vi "柱塞泵调试界面.vi"() -> ()   [LabVIEW 2016, in "质控单元.lvlib"]
uses:
  <vilib>/Utility/miscctls.llb/LVPointTypeDef.ctl
  <vilib>/Analysis/6fits.llb/Curve Fitting Criteria.ctl
  <vilib>/Utility/config.llb/Write Key (U32).vi
  <vilib>/Analysis/NI_AALPro.lvlib
  <vilib>/Utility/config.llb/NI_LVConfig.lvlib
panel:
  in  "B 5":dbl caption="B5"
  in  "K 5":dbl caption="K5"
  in  "柱塞泵5":bool
  out "关闭 2":bool=TRUE
  in  "柱塞泵4":bool
  in  "柱塞泵3":bool
  in  "柱塞泵2":bool
  in  "柱塞泵1":bool
  in  "注出体积选择":u16(ring) items=["0.1mL", "0.3mL", "0.5mL", "0.8mL", "1.0mL"]
  out "线性值":T1
  in  "读取":bool
  in  "写入":bool
  in  "柱塞泵枚举":enum16{"氨氮", "总磷", "总氮", "CODMn", "CODCr"}(ring)
  in  "启用计算":bool
  in  "标准体积 2":dbl
  in  "标准体积 3":dbl
  in  "实际体积 1":dbl
  in  "实际体积 2":dbl
  in  "实际体积 3":dbl
  in  "标准体积 4":dbl
  in  "实际体积 4":dbl
  in  "标准体积 5":dbl
  in  "实际体积 5":dbl
  in  "标准体积 1":dbl
  out "拟合方程":string
  out "r^2":dbl format="%_6g"
  in  "B 4":dbl caption="B4"
  in  "K 4":dbl caption="K4"
  in  "B 3":dbl caption="B3"
  in  "K 3":dbl caption="K3"
  in  "B 2":dbl caption="B2"
  in  "K 2":dbl caption="K2"
  in  "B":dbl caption="B1"
  in  "K":dbl caption="K1"
  in  "关闭":bool
  # "柱塞泵手动调试计算界面"
  # "柱塞泵启动控制"
  # "柱塞泵5点线性计算"
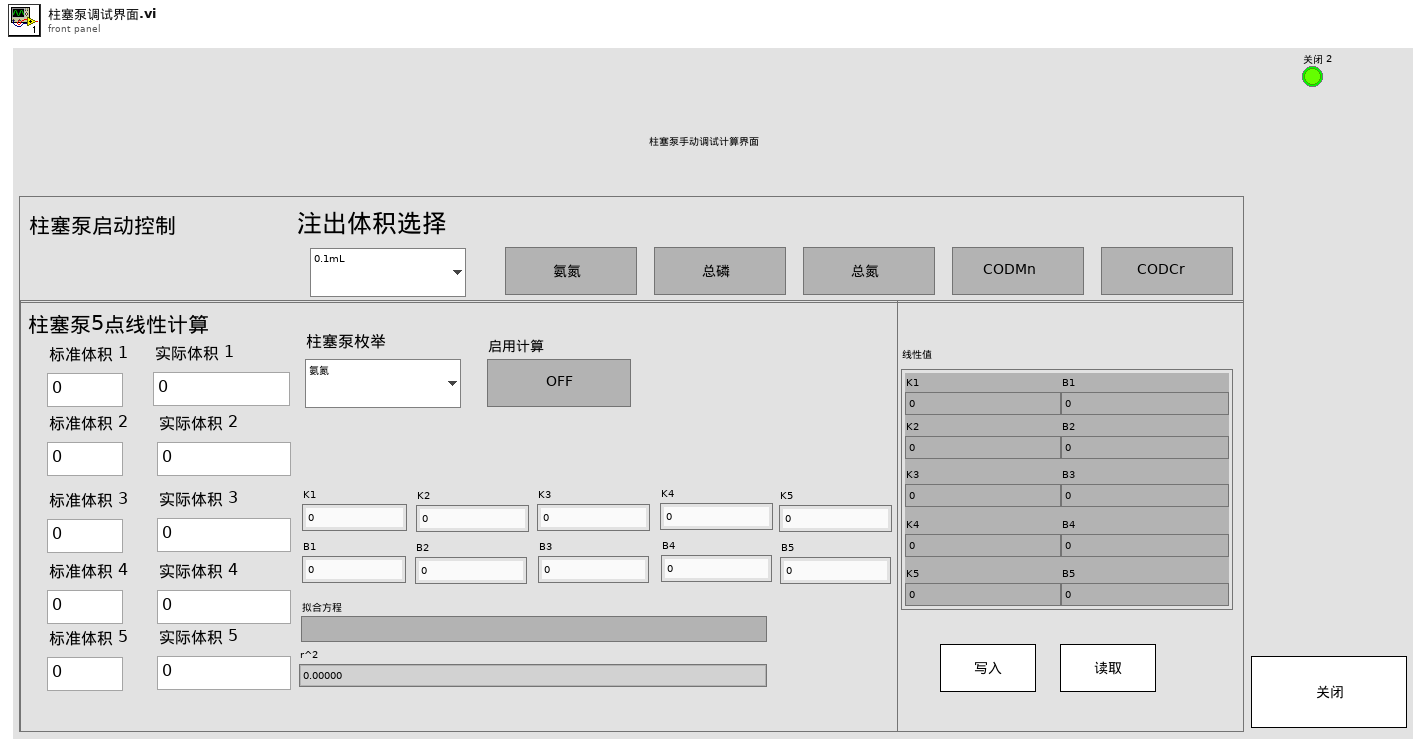
[diagram p1: front panel]
types:
  T1 = cluster{"K1":sgl, "B1":sgl, "K2":sgl, "B2":sgl, "K3":sgl, "B3":sgl, "K4":sgl, "B4":sgl, "K5":sgl, "B5":sgl}
  T2 = typedef "LVPointTypeDef.ctl" = cluster{"Horizontal":i16, "Vertical":i16}
  T3 = cluster{"氨氮":u8, "总磷":u8, "总氮":u8, "CODMn":u8, "CODCr":u8}
  T4 = typedef "NI_LVConfig.lvlib/Config Data RefNum.ctl" = refnum<k1>
  T5 = cluster{"数值":sgl, "数值":sgl, "数值":sgl, "数值":sgl, "数值":sgl, "数值":sgl, "数值":sgl, "数值":sgl, "数值":sgl, "数值":sgl}
  T6 = typedef "NI_AALPro.lvlib/Curve Fitting Criteria.ctl" = u16
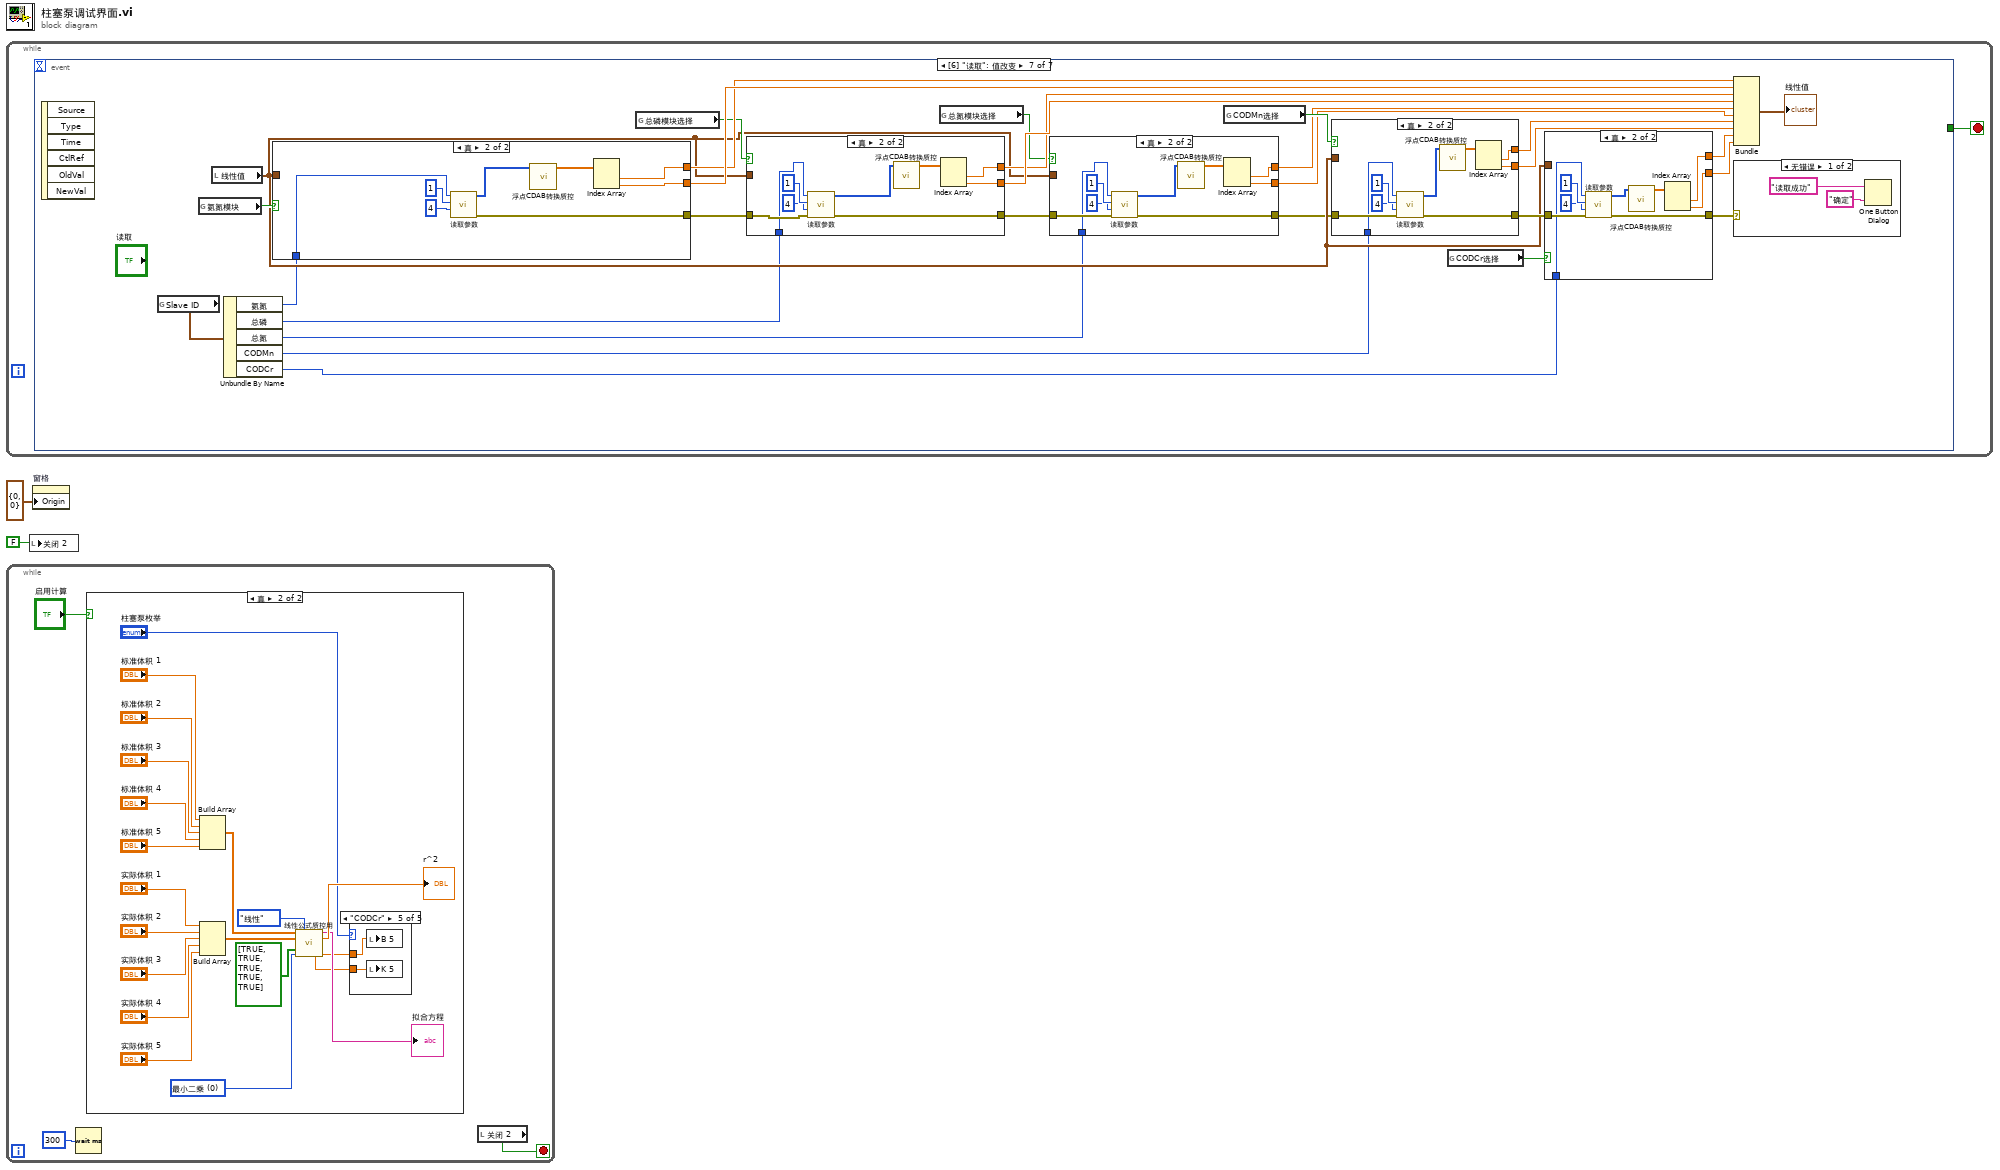
[diagram p0: block diagram]
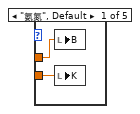
[diagram p3: hidden frame]
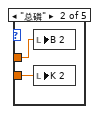
[diagram p4: hidden frame]
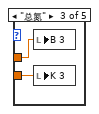
[diagram p5: hidden frame]
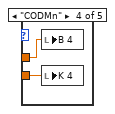
[diagram p6: hidden frame]
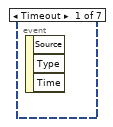
[diagram p7: hidden frame]
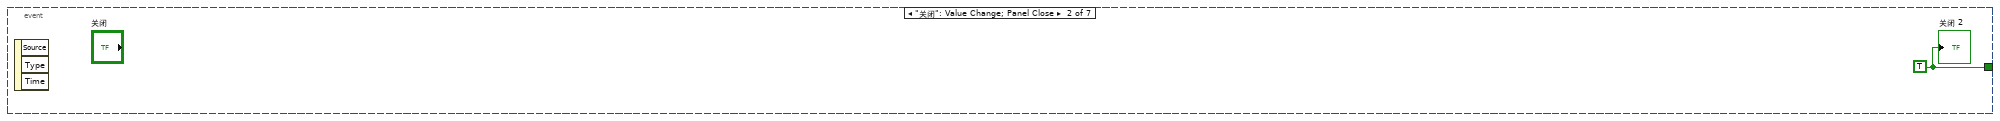
[diagram p8: hidden frame]
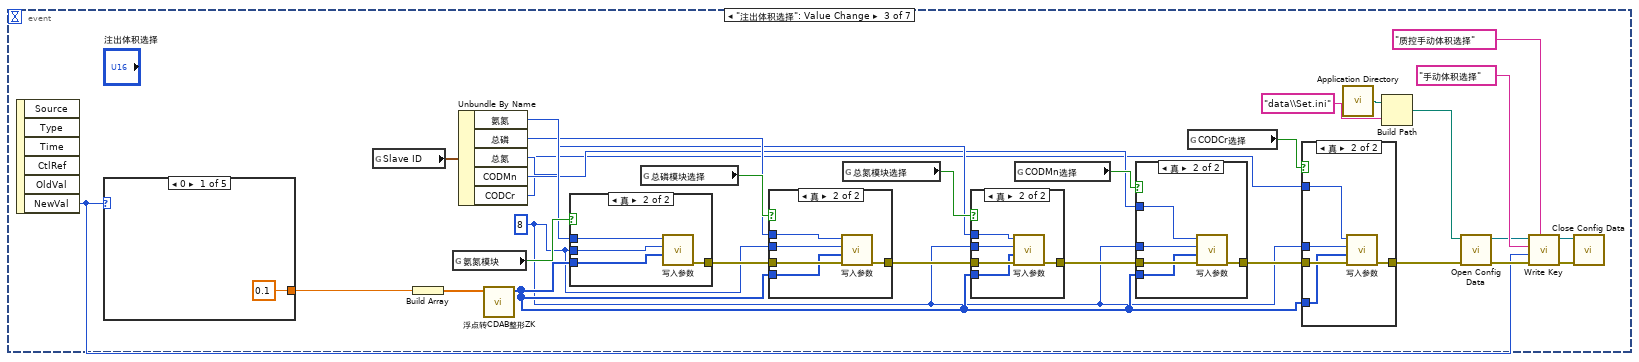
[diagram p9: hidden frame]
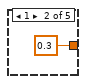
[diagram p15: hidden frame]
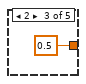
[diagram p16: hidden frame]
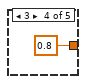
[diagram p17: hidden frame]
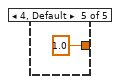
[diagram p18: hidden frame]
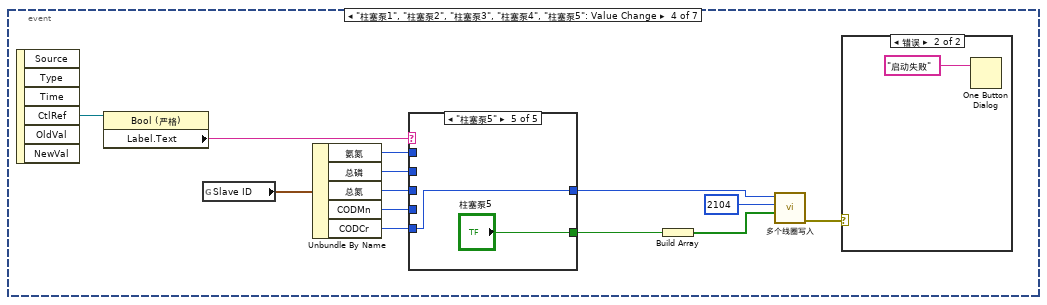
[diagram p19: hidden frame]
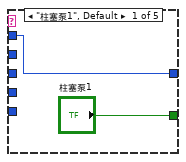
[diagram p20: hidden frame]
diagram:
  n1 = while {
    stop <- w3 stop-if-true
    n2 = event shown="[6] \"读取\": 值改变" {
      selector: _ -> [_ _ _ _ _ _ _]
      dyn-events: _ -> [_ _ _ _ _ _ _]
      timeout: _ -> [_ _ _ _ _ _ _]
      tunnel: [_ w4 _ _ _ _ _] -> w3
      event Timeout {
        n3 = event-data() -> ()  [unwired: 1 in, 3 out]
      }
      event "关闭": Value Change; Panel Close {
        w4 = TRUE ("关闭")
        n4 = event-data() -> ()  [unwired: 1 in, 3 out]
        "关闭 2" <- w4
      }
      event "注出体积选择": Value Change {
        w12 = u16 8 ("starting address")
        n5 = event-data() -> ("NewVal"=w16:u16)  [unwired: 1 in, 5 out]
        n6 = case shown="0" w16 {
          tunnel: [0.1 0.3 0.5 0.8 1.0] -> w18
          frame 0 {
          }
          frame 1 {
          }
          frame 2 {
          }
          frame 3 {
          }
          frame 4, Default {
          }
        }
        n7 = global read "断电保存全局.vi" "Slave ID"() -> (w10:T3)
        n8 = Build Array(w18) -> (w28:dbl[])
        n9 = global read "断电保存全局.vi" "氨氮模块"() -> (w31:bool)
        n10 = Unbundle By Name(w10) -> ("氨氮"=w9:u8, "总磷"=w8:u8, "总氮"=w7:u8, "CODMn"=w6:u8, "CODCr"=w5:u8)
        n11 = call "浮点转CDAB整形ZK.vi"("浮点数"=w28) -> ("CDAB整形输出"=w13:u16[])  [unwired: 10 in]
        n12 = case shown="真" w31 {
          tunnel: [_ w50] -> w17
          tunnel: w13 -> [_ w49]
          tunnel: w12 -> [_ w48]
          tunnel: w9 -> [_ w47]
          frame False {
          }
          frame True {
            n13 = call "写入参数.vi"("values"=w49, "starting address"=w48, "Slave ID"=w47) -> ("error out"=w50:errorcluster)  [unwired: 8 in]
          }
        }
        n14 = global read "断电保存全局.vi" "总磷模块选择"() -> (w32:bool)
        n15 = case shown="真" w32 {
          tunnel: w17 -> [w51 w56]
          tunnel: [w51 w55] -> w15
          tunnel: w12 -> [_ w54]
          tunnel: w13 -> [_ w53]
          tunnel: w8 -> [_ w52]
          frame False {
          }
          frame True {
            n16 = call "写入参数.vi"("Error in"=w56, "values"=w53, "starting address"=w54, "Slave ID"=w52) -> ("error out"=w55:errorcluster)  [unwired: 7 in]
          }
        }
        n17 = global read "断电保存全局.vi" "总氮模块选择"() -> (w11:bool)
        n18 = case shown="真" w11 {
          tunnel: w15 -> [w35 w40]
          tunnel: [w35 w39] -> w14
          tunnel: w12 -> [_ w38]
          tunnel: w13 -> [_ w37]
          tunnel: w7 -> [_ w36]
          frame False {
          }
          frame True {
            n19 = call "写入参数.vi"("Error in"=w40, "values"=w37, "starting address"=w38, "Slave ID"=w36) -> ("error out"=w39:errorcluster)  [unwired: 7 in]
          }
        }
        n20 = global read "断电保存全局.vi" "CODMn选择"() -> (w33:bool)
        n21 = case shown="真" w33 {
          tunnel: w14 -> [w57 w62]
          tunnel: w12 -> [_ w61]
          tunnel: [w57 w60] -> w29
          tunnel: w13 -> [_ w59]
          tunnel: w6 -> [_ w58]
          frame False {
          }
          frame True {
            n22 = call "写入参数.vi"("Error in"=w62, "values"=w59, "starting address"=w61, "Slave ID"=w58) -> ("error out"=w60:errorcluster)  [unwired: 7 in]
          }
        }
        n23 = global read "断电保存全局.vi" "CODCr选择"() -> (w34:bool)
        n24 = case shown="真" w34 {
          tunnel: w29 -> [w41 w46]
          tunnel: w12 -> [_ w45]
          tunnel: [w41 w44] -> w30
          tunnel: w13 -> [_ w43]
          tunnel: w5 -> [_ w42]
          frame False {
          }
          frame True {
            n25 = call "写入参数.vi"("Error in"=w46, "values"=w43, "starting address"=w45, "Slave ID"=w42) -> ("error out"=w44:errorcluster)  [unwired: 7 in]
          }
        }
        n26 = call <vilib>:"Application Directory.vi"() -> ("Application Directory"=w19:path)
        n27 = Build Path(base path=w19, name or relative path="data\\Set.ini" ("名称或相对路径")) -> (appended path=w21:path)
        n28 = call <vilib>:"Open Config Data.vi"("error in (no error)"=w30, "configuration file path"=w21) -> ("error out"=w25:errorcluster, "refnum"=w24:T4)  [unwired: 7 in, 1 out]
        n29 = call-poly <vilib>:"Write Key.vi"("section"="质控手动体积选择", "error in (no error)"=w25, "value"=w16, "key"="手动体积选择" ("section"), "refnum"=w24) -> ("error out"=w23:errorcluster, "refnum out"=w22:T4)  [unwired: 4 in, 1 out]
        n30 = call <vilib>:"Close Config Data.vi"("error in (no error)"=w23, "refnum"=w22) -> ()  [unwired: 8 in, 2 out]
      }
      event "柱塞泵1", "柱塞泵2", "柱塞泵3", "柱塞泵4", "柱塞泵5": Value Change {
        n31 = event-data() -> ("CtlRef"=w75:refnum<vi>)  [unwired: 1 in, 5 out]
        n32 = property class="Bool (严格)"(reference=w75) -> ("Label.Text"=w79:string)  [unwired: 1 in, 2 out]
        n33 = global read "断电保存全局.vi" "Slave ID"() -> (w73:T3)
        n34 = Unbundle By Name(w73) -> ("氨氮"=w72:u8, "总磷"=w71:u8, "总氮"=w70:u8, "CODMn"=w69:u8, "CODCr"=w68:u8)
        n35 = case shown="\"柱塞泵5\"" w79 {
          tunnel: [w81 w83 w85 w87 w89] -> w80
          tunnel: ["柱塞泵1" "柱塞泵2" "柱塞泵3" "柱塞泵4" "柱塞泵5"] -> w74
          tunnel: w72 -> [w81 _ _ _ _]
          tunnel: w71 -> [_ w83 _ _ _]
          tunnel: w70 -> [_ _ w85 _ _]
          tunnel: w69 -> [_ _ _ w87 _]
          tunnel: w68 -> [_ _ _ _ w89]
          frame "柱塞泵1", Default {
          }
          frame "柱塞泵2" {
          }
          frame "柱塞泵3" {
          }
          frame "柱塞泵4" {
          }
          frame "柱塞泵5" {
          }
        }
        n36 = Build Array(w74) -> (w77:bool[])
        n37 = call "多个线圈写入.vi"("values"=w77, "starting address"=u16 2104, "Slave ID"=w80) -> ("error out"=w78:errorcluster)  [unwired: 8 in]
        n38 = case shown="错误" w78 {
          frame No Error {
          }
          frame Error {
            n39 = One Button Dialog(message="启动失败" ("消息")) -> ()  [unwired: 1 in, 1 out]
          }
        }
      }
      event "标准体积 1", "实际体积 5", "标准体积 5", "实际体积 4", "标准体积 4", "实际体积 3", "实际体积 2", "实际体积 1", "标准体积 3", "标准体积 2", "线性值.K1", "线性值.B1", "线性值.K2", "线性值.B2", "线性值.K3", "线性值.B3", "线性值.K4", "线性值.B4", "线性值.K5", "线性值.B5": Mouse Down {
        n40 = event-data() -> ("CtlRef"=w95:refnum<vi>)  [unwired: 1 in, 7 out]
        n41 = property class="DigNum"(reference=w95) -> (reference out=w96:refnum<vi>, "Value"=w93:variant)  [unwired: 1 in, 1 out]
        n42 = Variant To Data(type=sgl 0.0 ("NewNumber"), Variant=w93) -> (data=w92:sgl)  [unwired: 1 in, 1 out]
        n43 = call "数字键盘.vi"("OldNumber"=w92) -> ("NewNumber"=w97:sgl)
        n44 = property class="DigNum"(reference=w96, "Val(Sgnl)"=w97) -> ()  [unwired: 1 in, 2 out]
      }
      event "写入": Value Change {
        n45 = event-data() -> ()  [unwired: 1 in, 6 out]
        n46 = control-ref of="柱塞泵枚举"() -> (w107:refnum<vi>)
        n47 = property class="Enum (严格)"(reference=w107) -> ("RingText.Text"=w106:string)  [unwired: 1 in, 2 out]
        n48 = Concatenate Strings("是否将K、B值写入" ("字符串"), w106, "？" ("字符串")) -> (w104:string)
        n49 = global read "断电保存全局.vi" "Slave ID"() -> (w103:T3)
        n50 = Unbundle By Name(w103) -> ("氨氮"=w102:u8, "总磷"=w101:u8, "总氮"=w100:u8, "CODMn"=w99:u8, "CODCr"=w98:u8)
        n51 = Two Button Dialog(message=w104) -> (T button?=w109:bool)  [unwired: 2 in]
        n52 = case shown="真" w109 {
          tunnel: w102 -> [_ w114]
          tunnel: w101 -> [_ w113]
          tunnel: w100 -> [_ w112]
          tunnel: w99 -> [_ w111]
          tunnel: w98 -> [_ w110]
          frame False {
          }
          frame True {
            n53 = local read "柱塞泵枚举"() -> (w115:enum16{"氨氮", "总磷", "总氮", "CODMn", "CODCr"})
            n54 = case shown="\"CODCr\"" w115 {
              tunnel: [w121 w132 w142 w152 w161] -> w116
              tunnel: w114 -> [w117 _ _ _ _]
              tunnel: w113 -> [_ w127 _ _ _]
              tunnel: w112 -> [_ _ w137 _ _]
              tunnel: w111 -> [_ _ _ w147 _]
              tunnel: w110 -> [_ _ _ _ w158]
              frame "氨氮", Default {
                w118 = 0 ("索引")
                n55 = Build Array("K", "B") -> (w123:dbl[])
                n56 = call "浮点转CDAB整形ZK.vi"("浮点数"=w123) -> ("CDAB整形输出"=w125:u16[])  [unwired: 10 in]
                n57 = Build Array(w118) -> (w124:i32[])
                n58 = Insert Into Array(array=w124, index=w118, new element=w125) -> (w126:i32[])
                n59 = call "写入参数.vi"("values"=w126, "starting address"=u16 1, "Slave ID"=w117) -> ("error out"=w121:errorcluster)  [unwired: 8 in]
              }
              frame "总磷" {
                w130 = 0 ("索引")
                n60 = Build Array("K 2", "B 2") -> (w134:dbl[])
                n61 = call "浮点转CDAB整形ZK.vi"("浮点数"=w134) -> ("CDAB整形输出"=w135:u16[])  [unwired: 10 in]
                n62 = Build Array(w130) -> (w133:i32[])
                n63 = Insert Into Array(array=w133, index=w130, new element=w135) -> (w136:i32[])
                n64 = call "写入参数.vi"("values"=w136, "starting address"=u16 1, "Slave ID"=w127) -> ("error out"=w132:errorcluster)  [unwired: 8 in]
              }
              frame "总氮" {
                w140 = 0 ("索引")
                n65 = Build Array("K 3", "B 3") -> (w145:dbl[])
                n66 = call "浮点转CDAB整形ZK.vi"("浮点数"=w145) -> ("CDAB整形输出"=w146:u16[])  [unwired: 10 in]
                n67 = Build Array(w140) -> (w144:i32[])
                n68 = Insert Into Array(array=w144, index=w140, new element=w146) -> (w143:i32[])
                n69 = call "写入参数.vi"("values"=w143, "starting address"=u16 1, "Slave ID"=w137) -> ("error out"=w142:errorcluster)  [unwired: 8 in]
              }
              frame "CODMn" {
                n70 = Build Array("K 4", "B 4") -> (w156:dbl[])
                n71 = call "浮点转CDAB整形ZK.vi"("浮点数"=w156) -> ("CDAB整形输出"=w157:u16[])  [unwired: 10 in]
                n72 = Build Array(0 ("背隙补偿步数")) -> (w154:i32[])
                n73 = Insert Into Array(array=w154, index=0 ("索引"), new element=w157) -> (w153:i32[])
                n74 = call "写入参数.vi"("values"=w153, "starting address"=u16 1, "Slave ID"=w147) -> ("error out"=w152:errorcluster)  [unwired: 8 in]
              }
              frame "CODCr" {
                n75 = Build Array("K 5", "B 5") -> (w167:dbl[])
                n76 = call "浮点转CDAB整形ZK.vi"("浮点数"=w167) -> ("CDAB整形输出"=w168:u16[])  [unwired: 10 in]
                n77 = Build Array(0 ("背隙补偿步数")) -> (w165:i32[])
                n78 = Insert Into Array(array=w165, index=0 ("索引"), new element=w168) -> (w164:i32[])
                n79 = call "写入参数.vi"("values"=w164, "starting address"=u16 1, "Slave ID"=w158) -> ("error out"=w161:errorcluster)  [unwired: 8 in]
              }
            }
            n80 = case shown="无错误" w116 {
              frame No Error {
                n81 = One Button Dialog(message="写入成功" ("消息"), button name ("OK")="确定" ("按钮名称（“确定”）")) -> ()  [unwired: 1 out]
              }
              frame Error {
                n82 = One Button Dialog(message="写入失败" ("消息"), button name ("OK")="确定" ("按钮名称（“确定”）")) -> ()  [unwired: 1 out]
              }
            }
          }
        }
      }
      event "读取": Value Change {
        n83 = event-data() -> ()  [unwired: 1 in, 6 out]
        n84 = global read "断电保存全局.vi" "Slave ID"() -> (w178:T3)
        n85 = global read "断电保存全局.vi" "氨氮模块"() -> (w200:bool)
        n86 = local read "线性值"() -> (w184:T1)
        n87 = Unbundle By Name(w178) -> ("氨氮"=w177:u8, "总磷"=w176:u8, "总氮"=w175:u8, "CODMn"=w174:u8, "CODCr"=w173:u8)
        n88 = case shown="真" w200 {
          tunnel: [errorcluster {"status"=FALSE, "code"=0, "source"=""} ("error out") w236] -> w191
          tunnel: [w229 w233] -> w192
          tunnel: [w228 w232] -> w193
          tunnel: w184 -> [w227 _]
          tunnel: w177 -> [_ w231]
          frame False {
            n89 = Unbundle By Name(w227) -> ("K1"=w229:sgl, "B1"=w228:sgl)
          }
          frame True {
            n90 = call "读取参数.vi"("Slave ID"=w231, "starting address"=u16 1, "quantity"=u16 4) -> ("values"=w235:u16[], "error out"=w236:errorcluster)  [unwired: 6 in]
            n91 = call "浮点CDAB转换质控.vi"("数组"=w235) -> ("数组 2"=w234:sgl[])  [unwired: 10 in]
            n92 = Index Array(array=w234) -> (element #1=w233:sgl, element #2=w232:sgl)  [unwired: 2 in]
          }
        }
        n93 = global read "断电保存全局.vi" "总磷模块选择"() -> (w190:bool)
        n94 = case shown="真" w190 {
          tunnel: w191 -> [w240 w251]
          tunnel: [w240 w250] -> w183
          tunnel: [w242 w247] -> w194
          tunnel: [w241 w246] -> w195
          tunnel: w184 -> [w239 _]
          tunnel: w176 -> [_ w243]
          frame False {
            n95 = Unbundle By Name(w239) -> ("K2"=w242:sgl, "B2"=w241:sgl)
          }
          frame True {
            n96 = call "读取参数.vi"("Slave ID"=w243, "starting address"=u16 1, "quantity"=u16 4, "Error in"=w251) -> ("values"=w249:u16[], "error out"=w250:errorcluster)  [unwired: 5 in]
            n97 = call "浮点CDAB转换质控.vi"("数组"=w249) -> ("数组 2"=w248:sgl[])  [unwired: 10 in]
            n98 = Index Array(array=w248) -> (element #1=w247:sgl, element #2=w246:sgl)  [unwired: 2 in]
          }
        }
        n99 = global read "断电保存全局.vi" "总氮模块选择"() -> (w185:bool)
        n100 = case shown="真" w185 {
          tunnel: w183 -> [w202 w213]
          tunnel: [w202 w212] -> w182
          tunnel: [w204 w209] -> w181
          tunnel: [w203 w208] -> w180
          tunnel: w184 -> [w201 _]
          tunnel: w175 -> [_ w205]
          frame False {
            n101 = Unbundle By Name(w201) -> ("K3"=w204:sgl, "B3"=w203:sgl)
          }
          frame True {
            n102 = call "读取参数.vi"("Slave ID"=w205, "starting address"=u16 1, "quantity"=u16 4, "Error in"=w213) -> ("values"=w211:u16[], "error out"=w212:errorcluster)  [unwired: 5 in]
            n103 = call "浮点CDAB转换质控.vi"("数组"=w211) -> ("数组 2"=w210:sgl[])  [unwired: 10 in]
            n104 = Index Array(array=w210) -> (element #1=w209:sgl, element #2=w208:sgl)  [unwired: 2 in]
          }
        }
        n105 = global read "断电保存全局.vi" "CODMn选择"() -> (w199:bool)
        n106 = case shown="真" w199 {
          tunnel: w182 -> [w253 w264]
          tunnel: [w255 w261] -> w186
          tunnel: [w254 w260] -> w187
          tunnel: [w253 w257] -> w196
          tunnel: w184 -> [w252 _]
          tunnel: w174 -> [_ w256]
          frame False {
            n107 = Unbundle By Name(w252) -> ("K4"=w255:sgl, "B4"=w254:sgl)
          }
          frame True {
            n108 = call "读取参数.vi"("Slave ID"=w256, "starting address"=u16 1, "quantity"=u16 4, "Error in"=w264) -> ("values"=w263:u16[], "error out"=w257:errorcluster)  [unwired: 5 in]
            n109 = call "浮点CDAB转换质控.vi"("数组"=w263) -> ("数组 2"=w262:sgl[])  [unwired: 10 in]
            n110 = Index Array(array=w262) -> (element #1=w261:sgl, element #2=w260:sgl)  [unwired: 2 in]
          }
        }
        n111 = global read "断电保存全局.vi" "CODCr选择"() -> (w198:bool)
        n112 = case shown="真" w198 {
          tunnel: w196 -> [w215 w226]
          tunnel: [w217 w223] -> w188
          tunnel: [w216 w222] -> w189
          tunnel: [w215 w219] -> w197
          tunnel: w184 -> [w214 _]
          tunnel: w173 -> [_ w218]
          frame False {
            n113 = Unbundle By Name(w214) -> ("K5"=w217:sgl, "B5"=w216:sgl)
          }
          frame True {
            n114 = call "读取参数.vi"("Slave ID"=w218, "starting address"=u16 1, "quantity"=u16 4, "Error in"=w226) -> ("values"=w225:u16[], "error out"=w219:errorcluster)  [unwired: 5 in]
            n115 = call "浮点CDAB转换质控.vi"("数组"=w225) -> ("数组 2"=w224:sgl[])  [unwired: 10 in]
            n116 = Index Array(array=w224) -> (element #1=w223:sgl, element #2=w222:sgl)  [unwired: 2 in]
          }
        }
        n117 = Bundle("数值"=w192, "数值"=w193, "数值"=w194, "数值"=w195, "数值"=w181, "数值"=w180, "数值"=w186, "数值"=w187, "数值"=w188, "数值"=w189) -> (→"线性值":T5)  [unwired: 1 in]
        n118 = case shown="无错误" w197 {
          frame No Error {
            n119 = One Button Dialog(message="读取成功" ("消息"), button name ("OK")="确定" ("按钮名称（“确定”）")) -> ()  [unwired: 1 out]
          }
          frame Error {
            n120 = One Button Dialog(message="读取失败" ("消息"), button name ("OK")="确定" ("按钮名称（“确定”）")) -> ()  [unwired: 1 out]
          }
        }
      }
    }
  }
  n121 = while {
    stop <- w270 stop-if-true
    n122 = Wait (ms)(milliseconds to wait=u32 300 ("等待时间（毫秒）")) -> ()  [unwired: 1 out]
    n123 = case shown="真" "启用计算" {
      frame False {
      }
      frame True {
        w288 = T6 0 items=["最小二乘", "最小绝对残差", "Bisquare"] ("method")
        n124 = Build Array("标准体积 1", "标准体积 2", "标准体积 3", "标准体积 4", "标准体积 5") -> (w285:dbl[])
        n125 = Build Array("实际体积 1", "实际体积 2", "实际体积 3", "实际体积 4", "实际体积 5") -> (w286:dbl[])
        n126 = call "线性公式质控用.vi"("标液浓度"=w285, "模型"=enum32{"线性", "多项式"}."线性", "监测浓度"=w286, "启用"=bool[] [TRUE, TRUE, TRUE, TRUE, TRUE], "method"=w288) -> ("拟合方程"=→"拟合方程":string, "r^2"=→"r^2":dbl, "slope"=w274:dbl, "intercept"=w273:dbl)  [unwired: 6 in, 1 out]
        n127 = case shown="\"CODCr\"" "柱塞泵枚举" {
          tunnel: w274 -> [w292 w295 w296 w299 w301]
          tunnel: w273 -> [w293 w294 w297 w298 w300]
          frame "氨氮", Default {
            n128 = local write "B"(w293) -> ()
            n129 = local write "K"(w292) -> ()
          }
          frame "总磷" {
            n130 = local write "B 2"(w294) -> ()
            n131 = local write "K 2"(w295) -> ()
          }
          frame "总氮" {
            n132 = local write "B 3"(w297) -> ()
            n133 = local write "K 3"(w296) -> ()
          }
          frame "CODMn" {
            n134 = local write "B 4"(w298) -> ()
            n135 = local write "K 4"(w299) -> ()
          }
          frame "CODCr" {
            n136 = local write "B 5"(w300) -> ()
            n137 = local write "K 5"(w301) -> ()
          }
        }
      }
    }
    n138 = local read "关闭 2"() -> (w270:bool)
  }
  n139 = local write "关闭 2"(FALSE ("关闭 2")) -> ()
  n140 = property on="窗格" class="Pane"("Origin"=T2 {"Horizontal"=0, "Vertical"=0} ("原点")) -> ()  [unwired: 2 in, 2 out]
